vi "Read.vi"(7 "Slave Address":u8, 8 "Error In":errorcluster, 10 "Count":i32, 11 "AD2 I2C In":refnum<class "AD2 I2C.lvclass">=refnum) -> (0 "Error Out":errorcluster, 2 "Data":u8[](array[numeric]), 3 "AD2 I2C Out":refnum<class "AD2 I2C.lvclass">)   [LabVIEW 2020, in "lv_i2c_ad2.lvlib" / "AD2 I2C.lvclass"]
uses:
  AD2 I2C.lvclass
  AD2 I2C.lvclass/AD2 I2C.ctl
  <vilib>/miidas/lv_i2c_ad2/lv_waveforms_toolkit.lvlib
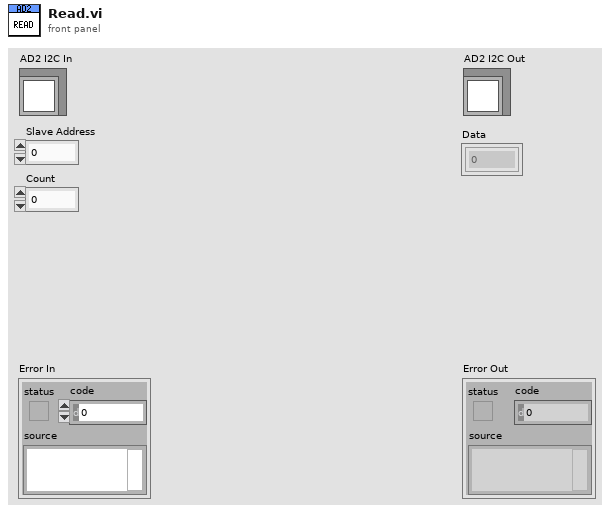
[diagram p1: front panel]
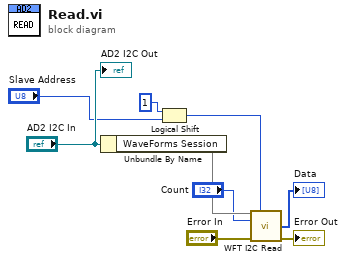
[diagram p0: block diagram]
diagram:
  n1 = Unbundle By Name("AD2 I2C In") -> ("WaveForms Session"=w7)
  n2 = Logical Shift(y=i16 1, x="Slave Address") -> (x << y=w1:u8)
  n3 = call <vilib>:"WFT I2C Read.vi"("WaveForms Session In"=w7, "adr8Bits"=w1, "cRx"="Count", "Error In"="Error In") -> ("rgbRx"=→"Data":u8[], "Error Out"=→"Error Out":errorcluster)  [unwired: 7 in, 3 out]
  "AD2 I2C Out" <- "AD2 I2C In"
